vi "SpectToWaveform.vi"() -> ()   [LabVIEW 2014]
uses:
  <vilib>/Utility/file.llb/Read From Spreadsheet File (DBL).vi
panel:
  out "RL Spectrum":cluster{"Array":dbl[], "Array":dbl[]}[](array[cluster])
  out "XY Graph":cluster{dbl[], dbl[]}[](graph)
  out "Spectrun File in":string="mySP2-40-Spectrum mar-13-2021 Time 10-05.spt"
  out "Total Specs":i32=105
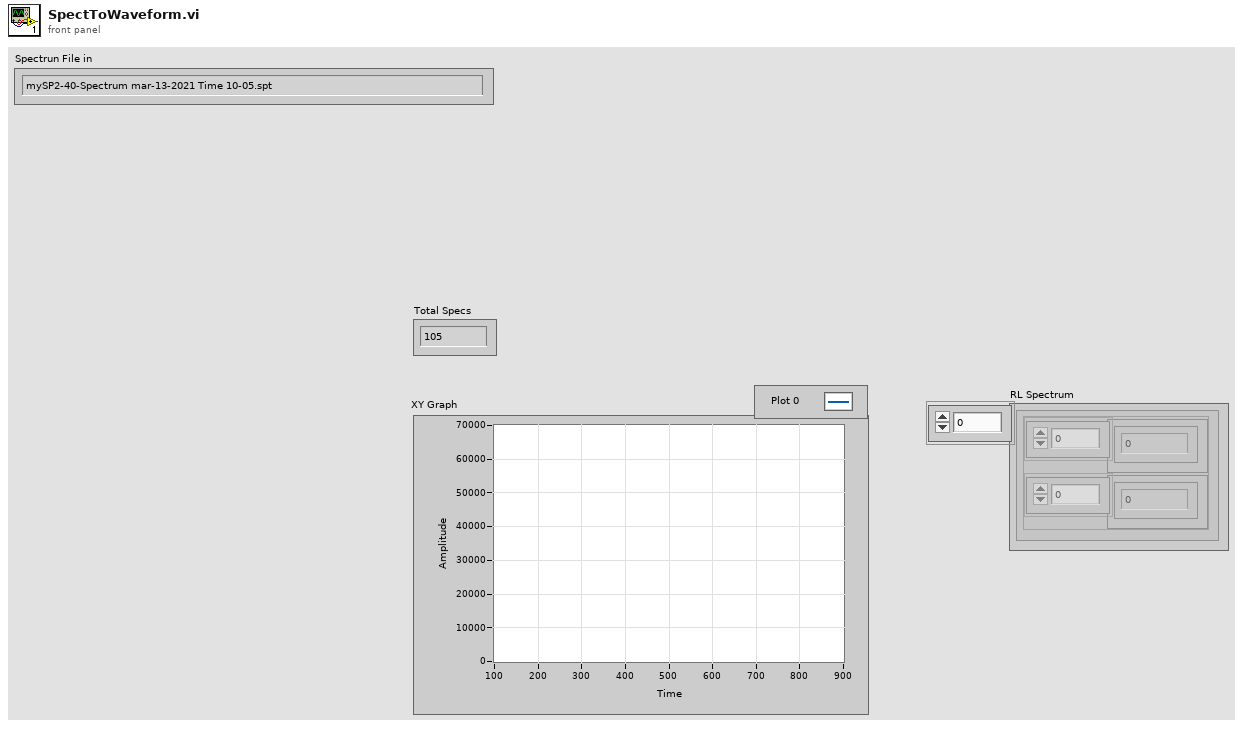
[diagram p1: front panel]
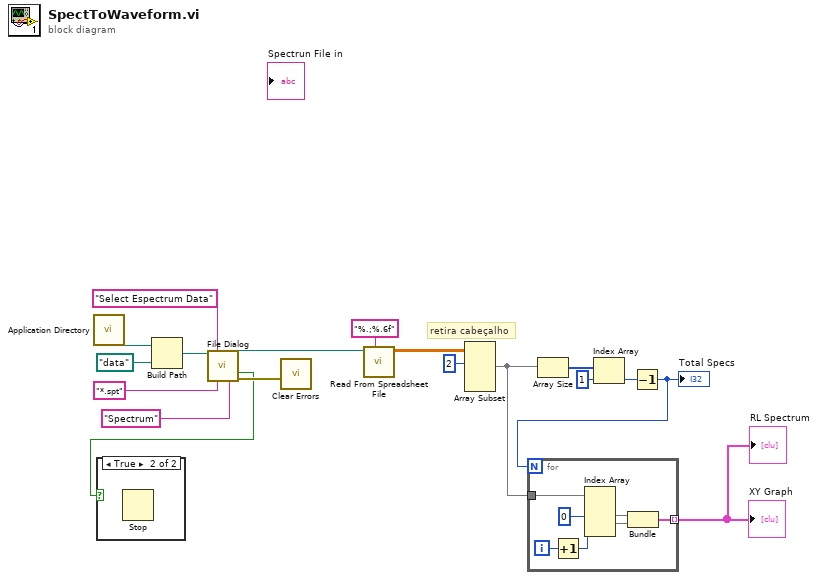
[diagram p0: block diagram]
diagram:
  # "retira cabeçalho"
  n1 = call <vilib>:"Application Directory.vi"() -> ("Application Directory"=w14:path)
  n2 = Build Path(base path=w14, name or relative path=path "data") -> (appended path=w13:path)
  n3 = call "File Dialog"("start path"=w13, "prompt"="Select Espectrum Data", "pattern (all files)"="*.spt", "pattern label"="Spectrum") -> ("selected path"=w5:path, "cancelled"=w4:bool, "error out"=w12:errorcluster)  [unwired: 8 in, 1 out]
  n4 = case shown="True" w4 {
    frame False {
    }
    frame True {
      n5 = Stop() -> ()  [unwired: 1 in]
    }
  }
  n6 = call <vilib>:"Clear Errors.vi"("error in (no error)"=w12) -> ()  [unwired: 5 in, 2 out]
  n7 = call-poly <vilib>:"Read From Spreadsheet File.vi"("format (%.3f)"="%.;%.6f", "file path (dialog if empty)"=w5) -> ("all rows"=w9:dbl[][])  [unwired: 5 in, 4 out]
  n8 = Array Subset(array=w9, index (row)=2 ("index")) -> (w2:dbl[][])  [unwired: 3 in]
  n9 = Array Size(array=w2) -> (size(s)=w8:i32[])
  n10 = Index Array(array=w8, index=1) -> (element=w6:i32)
  n11 = Decrement(x=w6) -> (x-1=w3:i32)
  "Total Specs" <- w3
  n12 = for {
    N: w3 -> [_]
    tunnel: w2 -> [w25]
    tunnel: [w21] -> w1 mode=indexing
    i -> [w20]
    n13 = Increment(x=w20) -> (x+1=w19:i32)
    n14 = Index Array(array=w25, index (col) #1=0 ("index (row)"), index (col) #2=w19) -> (element #1=w23:dbl[], element #2=w22:dbl[])  [unwired: 2 in]
    n15 = Bundle(w23, w22) -> (w21:cluster{dbl[], dbl[]})  [unwired: 1 in]
  }
  "XY Graph" <- w1
  "RL Spectrum" <- w1
